vi "Main.vi"() -> ()   [LabVIEW 2014]
uses:
  <userlib>/ROS for LabVIEW Software/ROS/Code/Console/Servers/ServerSubs/TopicDef.ctl
  <userlib>/ROS for LabVIEW Software/ROS/Code/SubVIs/_ROSDirection.ctl
  <userlib>/ROS for LabVIEW Software/ROS/MessageBuilding/std_msgs/subs/stringScalar.vi
panel:
  in  "I said:":string="Hello world!"
  out "error out":errorcluster
  in  "stop":bool
  # "Overview: The myRIO Project template acquires acceleration data from the onboard accelerometer and displays the changes of acceleration values in a waveform chart.\nInstructions:\n1. Check the myRIO target IP Address in the project and make sure the target IP Address is correct. \n2. Run the VI."
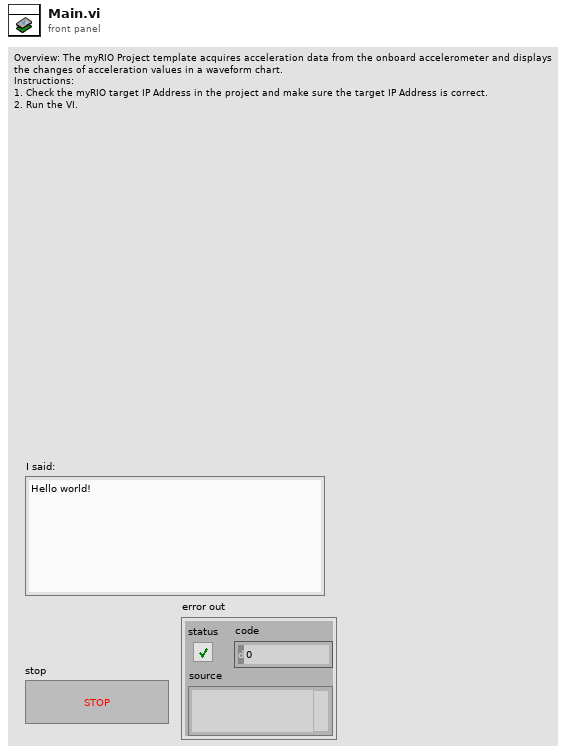
[diagram p1: front panel]
types:
  T1 = typedef "TopicDef.ctl" = cluster{"Topic":string, "Type":string, "Action":T2, "Update (ms)":u16, "queue size":u16}
  T2 = typedef "_ROSDirection.ctl" = enum16{"Node", "Publisher", "Subscriber", "ServiceClient", "ServiceProvider"}
  T3 = typedef "_ROSControl.ctl" = cluster{"topic port":u16, "Node":string, "topic":string, "type":string, "node port":u16, "error ":errorcluster, "Direction":T2, "Update (ms)":u16, "FIFO size":u16}
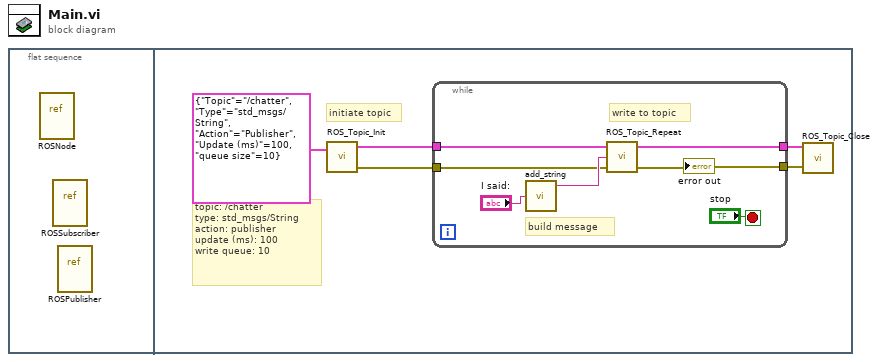
[diagram p0: block diagram]
diagram:
  n1 = flat-sequence {
    frame #0 {
      n2 = vi-ref <userlib>:"ROSNode.vi"() -> ()  [unwired: 1 out]
      n3 = vi-ref <userlib>:"ROSSubscriber.vi"() -> ()  [unwired: 1 out]
      n4 = vi-ref <userlib>:"ROSPublisher.vi"() -> ()  [unwired: 1 out]
    }
    frame #1 {
      # "initiate topic"
      # "topic: /chatter\ntype: std_msgs/String\naction: publisher\nupdate (ms): 100\nwrite queue: 10"
      n5 = call <userlib>:"ROS_Topic_Init.vi"("Definitions"=T1 {"Topic"="/chatter", "Type"="std_msgs/String", "Action"=enum."Publisher", "Update (ms)"=100, "queue size"=10}) -> ("ROS out"=w4:T3, "error out"=w3:errorcluster)  [unwired: 2 in]
      n6 = while {
        tunnel: w4 -> [w12]
        tunnel: w3 -> [w9]
        tunnel: [w7] -> w2
        tunnel: [w6] -> w1
        stop <- "stop" stop-if-true
        # "build message"
        # "write to topic"
        n7 = call-poly <userlib>:"add_string.vi"("String"="I said:") -> ("msg out"=w10:string)  [unwired: 4 in]
        n8 = call <userlib>:"ROS_Topic_Repeat.vi"("error in (no error)"=w9, "Msg in"=w10, "ROS in"=w12) -> ("error out"=w6:errorcluster, "ROS out"=w7:T3)  [unwired: 1 in]
        "error out" <- w6
      }
      n9 = call <userlib>:"ROS_Topic_Close.vi"("error in"=w1, "ROS in"=w2) -> ()  [unwired: 2 in, 1 out]
    }
  }
